vi "WPI_ServoSetPosition.vi"(8 "error in (no error)":errorcluster, 10 "Position":dbl, 11 "ServoDeviceRef":T1={"DeviceStatus"={"status"=FALSE, "code"=0, "source"=""}, "PWM Channel"=enum."Invalid", "DeadBand"={"Name"="", "maxPositivePwm"=0, "minPositivePwm"=0, "centerPwm"=0, "maxNegativePwm"=0, "minNegativePwm"=0, "angularRange"=0}}) -> (0 "error out":errorcluster, 3 "ServoDeviceRef":T1={"DeviceStatus"={"status"=FALSE, "code"=0, "source"=""}, "PWM Channel"=enum."Invalid", "DeadBand"={"Name"="", "maxPositivePwm"=0, "minPositivePwm"=0, "centerPwm"=0, "maxNegativePwm"=0, "minNegativePwm"=0, "angularRange"=0}})   [LabVIEW 2017]
doc: "Specifies the position of the servo you specify.\n\nThis software is licensed. Open the labview\\readme\\WPI Robotics Library Open Source License.txt file for more information."
uses:
  <vilib>/Rock Robotics/WPI/PWM/Servo/WPI_ServoDeviceRef.ctl
  <vilib>/Rock Robotics/SystemInterfaces/DIO/FPGA_DIOPWMChannel.ctl
  <vilib>/Rock Robotics/WPI/PWM/WPI_PWMDeadband.ctl
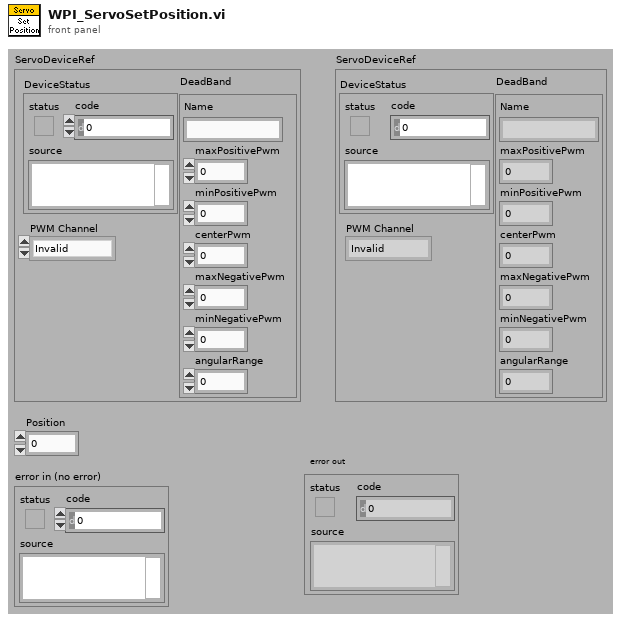
[diagram p1: front panel]
types:
  T1 = typedef "WPI_ServoDeviceRef.ctl" = cluster{"DeviceStatus":errorcluster, "PWM Channel":T2, "DeadBand":T3}
  T2 = typedef "FPGA_DIOPWMChannel.ctl" = enum8{"PWM 0", "PWM 1", "PWM 2", "PWM 3", "PWM 4", "PWM 5", "PWM 6", "PWM 7", "PWM 8", "PWM 9", "PWM MXP 0", "PWM MXP 1", "PWM MXP 2", "PWM MXP 3", "PWM MXP 4", "PWM MXP 5", "PWM MXP 6", "PWM MXP 7", "PWM MXP 8", "PWM MXP 9", "Invalid"}
  T3 = typedef "WPI_PWMDeadband.ctl" = cluster{"Name":string, "maxPositivePwm":i32, "minPositivePwm":i32, "centerPwm":i32, "maxNegativePwm":i32, "minNegativePwm":i32, "angularRange":u16}
  T4 = typedef "WPI_PWMDeviceRef.ctl" = cluster{"DeviceStatus":errorcluster, "PWM Channel":T2}
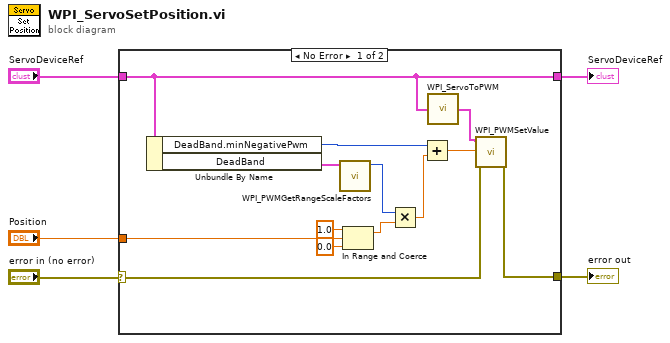
[diagram p0: block diagram]
diagram:
  n1 = case shown="No Error" "error in (no error)" {
    selector: "error in (no error)" -> [w7 w20]
    tunnel: "ServoDeviceRef" -> [w8 w19]
    tunnel: [w8 w19] -> w4
    tunnel: "Position" -> [w18 _]
    tunnel: [w6 w20] -> w2
    frame No Error {
      n2 = Unbundle By Name(w8) -> ("DeadBand.minNegativePwm"=w17:i32, "DeadBand"=w10:T3)
      n3 = call <vilib>:"WPI_PWMGetRangeScaleFactors.vi"("DeadBand"=w10) -> ("fullRangeScaleFactor"=w11:i32)  [unwired: 10 out]
      n4 = In Range and Coerce(upper limit=1.0, x=w18, lower limit=0.0) -> (coerced(x)=w14:dbl)  [unwired: 1 out]
      n5 = Multiply(x=w11, y=w14) -> (x*y=w13:dbl)
      n6 = Add(x=w17, y=w13) -> (x+y=w12:dbl)
      n7 = call <vilib>:"WPI_ServoToPWM.vi"("ServoDeviceRef"=w8) -> ("PWMDeviceRef"=w9:T4)
      n8 = call <vilib>:"WPI_PWMSetValue.vi"("error in (no error)"=w7, "Value"=w12, "PWMDeviceRef"=w9) -> ("error out"=w6:errorcluster)  [unwired: 1 in, 7 out]
    }
    frame Error {
    }
  }
  "ServoDeviceRef" <- w4
  "error out" <- w2
